vi "2DRangefinderMerge.vi"() -> ()   [LabVIEW 2017]
uses:
  <vilib>/robotics/Controls/2D Rangefinder/NI_Robotics_2D Rangefinder.xctl
panel:
  out "Rangefinder Indicator":cluster{"angle":dbl[], "distance":dbl[][]}(xcontrol)
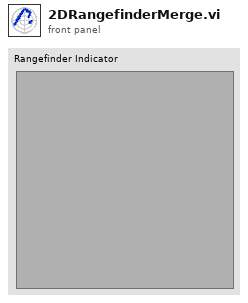
[diagram p1: front panel]
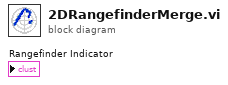
[diagram p0: block diagram]
diagram:
